vi "Set Travel Speed.vi"(8 "error in (no error)":errorcluster, 9 "Speed":dbl format="%.2f", 10 "Speed Units":T1, 11 "ESM303 in":refnum<class "ESM303.lvclass">) -> (0 "error out":errorcluster, 3 "ESM303 out":refnum<class "ESM303.lvclass">)   [LabVIEW 2018, in "ESM303.lvlib" / "ESM303.lvclass"]
uses:
  ESM303.lvclass
  builds/Force Test Stand/Force Test Stand/Force Test Stand.lvlibp/Custom Controls/Speed Units.ctl
  builds/Force Test Stand/Force Test Stand/Force Test Stand.lvlibp/Force Test Stand.lvclass
  C:/Projects/LabVIEW/In-Progress/Jose Rivero-Diaz/builds/Force Test Stand/Force Test Stand/Force Test Stand.lvlibp/Force Test Stand.lvclass
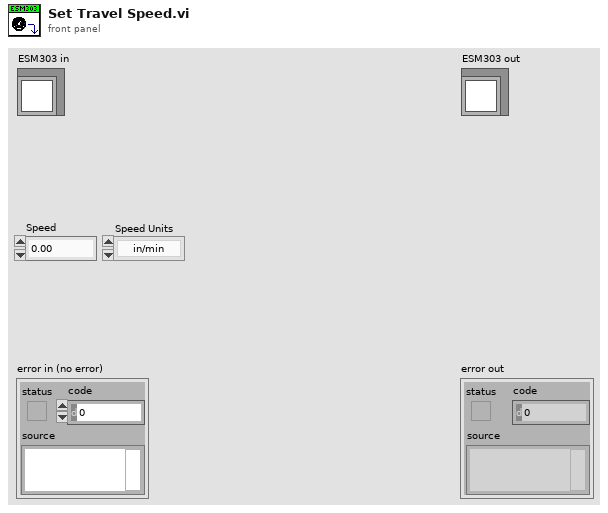
[diagram p1: front panel]
types:
  T1 = typedef "Force Test Stand.lvlibp/Force Test Stand.lvclass/Speed Units.ctl" = enum16{"in/min", "mm/min"}
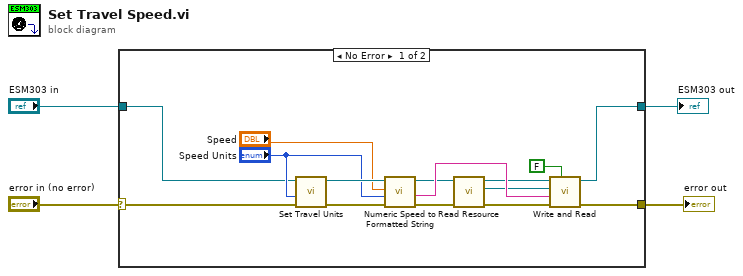
[diagram p0: block diagram]
diagram:
  n1 = case shown="No Error" "error in (no error)" {
    selector: "error in (no error)" -> [w8 w21]
    tunnel: [w19 w21] -> w3
    tunnel: [w18 w20] -> w2
    tunnel: "ESM303 in" -> [w11 w20]
    frame No Error {
      n2 = call-dynamic "Set Travel Units.vi"("error in (no error)"=w8, "Speed Units"="Speed Units", "ESM303 in"=w11) -> ("error out"=w15:errorcluster, "ESM303 out"=w16:refnum<class "ESM303.lvclass">)  [unwired: 7 in]
      n3 = call "Numeric Speed to Formatted String.vi"("error in (no error)"=w15, "Speed Units"="Speed Units", "Speed"="Speed", "ESM303 in"=w16) -> ("error out"=w10:errorcluster, "Formatted Speed String"=w12:string, "ESM303 out"=w9:refnum<class "ESM303.lvclass">)  [unwired: 5 in]
      n4 = call "Read Resource.vi"("error in (no error)"=w10, "Force Test Stand in"=w9) -> ("error out"=w7:errorcluster, "Resource"=w5:refnum<visa-resource-name>, "Force Test Stand out"=w6:refnum<class "ESM303.lvclass">)  [unwired: 7 in]
      n5 = call "Write and Read.vi"("Write & Read"=FALSE, "error in (no error)"=w7, "Command"=w12, "VISA Refnum in"=w5, "ESM303 in"=w6) -> ("error out"=w19:errorcluster, "ESM303 out"=w18:refnum<class "ESM303.lvclass">)  [unwired: 4 in, 1 out]
    }
    frame Error {
    }
  }
  "error out" <- w3
  "ESM303 out" <- w2
